vi "Untitled 39.vi"() -> ()   [LabVIEW 2020]
panel:
  out "error out":errorcluster
  in  "file path":path
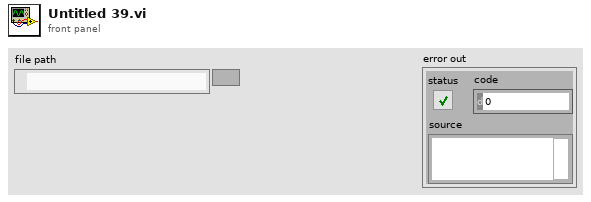
[diagram p1: front panel]
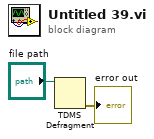
[diagram p0: block diagram]
diagram:
  n1 = TDMS Defragment(7:"file path") -> (0:→"error out":errorcluster)  [unwired: 1 in]
